vi "(SubVI)_Reset_AOs_before_turnoff.vi"(2 "data":dbl[](array[numeric]) format="%0.2f", 3 "Sti. Galvo AOs and Laser Driver AO Task Out":refnum<k21>, 4 "Sti. Galvo AOs and Laser Driver AO Chns":tag) -> (0 "error out":errorcluster, 1 "task out":refnum<k21>)   [LabVIEW 2019]
uses:
  <vilib>/DAQmx/write.llb/DAQmx Write (Analog 1D DBL NChan 1Samp).vi
  <vilib>/DAQmx/create/channels.llb/DAQmx Create Channel (AO-Voltage-Basic).vi
  <vilib>/DAQmx/miscellaneous.llb/DAQmx Fill In Error Info.vi
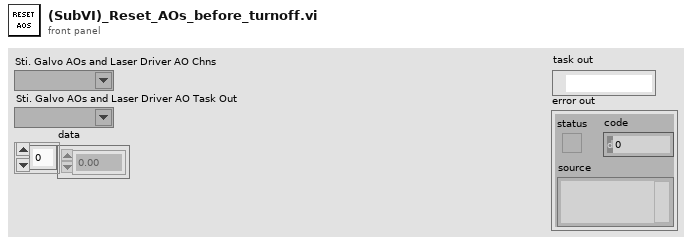
[diagram p1: front panel]
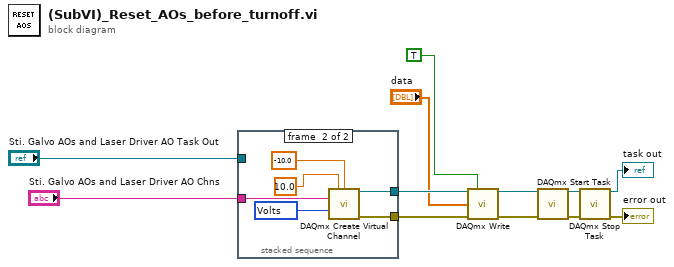
[diagram p0: block diagram]
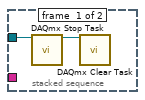
[diagram p2: hidden frame]
diagram:
  n1 = stacked-sequence {
    tunnel: "Sti. Galvo AOs and Laser Driver AO Task Out" -> [w14 _]
    tunnel: "Sti. Galvo AOs and Laser Driver AO Chns" -> [_ w17]
    tunnel: [_ w16] -> w11
    tunnel: [_ w15] -> w12
    frame #0 {
      n2 = call <vilib>:"DAQmx Stop Task.vi"("task/channels in"=w14) -> ("task out"=w13:refnum<k21>)  [unwired: 13 in, 1 out]
      n3 = call <vilib>:"DAQmx Clear Task.vi"("task in"=w13) -> ()  [unwired: 14 in, 1 out]
    }
    frame #1 {
      w18 = 10348 items=["Volts"=10348, "From Custom Scale"=10065] ("units")
      n4 = call-poly <vilib>:"DAQmx Create Virtual Channel.vi"("maximum value"=10.0, "minimum value"=-10.0, "physical channels"=w17, "units"=w18) -> ("task out"=w16:refnum<k21>, "error out"=w15:errorcluster)  [unwired: 5 in, 5 out]
    }
  }
  n5 = call-poly <vilib>:"DAQmx Write.vi"("task/channels in"=w11, "auto start"=TRUE, "data"="data", "error in"=w12) -> ("task out"=w6:refnum<k21>, "error out"=w8:errorcluster)  [unwired: 10 out]
  n6 = call <vilib>:"DAQmx Start Task.vi"("task/channels in"=w6, "error in"=w8) -> ("task out"=w9:refnum<k21>, "error out"=w10:errorcluster)  [unwired: 12 in]
  n7 = call <vilib>:"DAQmx Stop Task.vi"("task/channels in"=w9, "error in"=w10) -> ("task out"=→"task out":refnum<k21>, "error out"=→"error out":errorcluster)  [unwired: 12 in]
